vi "findRangeBearing.vi"(9 "X":dbl[](array[numeric]), 10 "ly":dbl, 11 "lx":dbl) -> (2 "tt":dbl, 3 "rr":dbl)   [LabVIEW 2009, in "LV_SLAM.lvlib"]
uses:
  LV_SLAM.lvlib
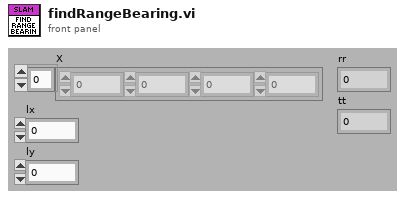
[diagram p1: front panel]
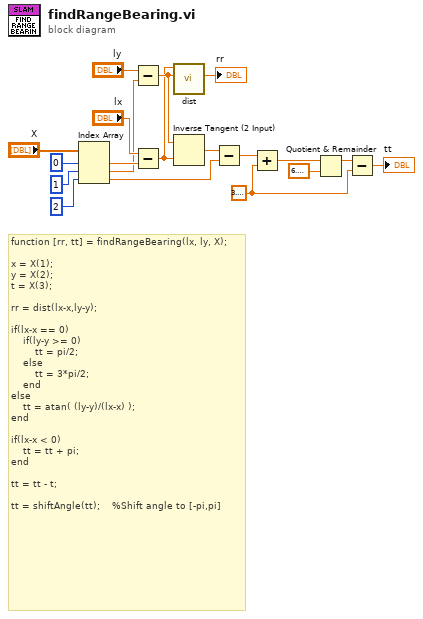
[diagram p0: block diagram]
diagram:
  w2 = 3.141592653589793
  # "function [rr, tt] = findRangeBearing(lx, ly, X);\n\nx = X(1);\ny = X(2);\nt = X(3);\n\nrr = dist(lx-x,ly-y);\n\nif(lx-x == 0)\n    if(ly-y >= 0)\n        tt = pi/2;\n    else\n        tt = 3*pi/2;\n    end\nelse\n    tt = atan( (ly-y)/(lx-x) );\nend\n\nif(lx-x < 0)\n    tt = tt + pi;\nend\n\ntt = tt - t;    \n\ntt = shiftAngle(tt);    %Shift angle to [-pi,pi]"
  n1 = Index Array(array="X", index #1=0 ("index"), index #2=1 ("index"), index #3=2 ("index")) -> (element #1=w14:dbl, element #2=w12:dbl, element #3=w7:dbl)
  n2 = Subtract(x="ly", y=w12) -> (x-y=w10:dbl)
  n3 = Subtract(x="lx", y=w14) -> (x-y=w9:dbl)
  n4 = call "dist.vi"("y"=w10, "x"=w9) -> ("d"=→"rr":dbl)  [unwired: 9 in]
  n5 = Inverse Tangent (2 Input)(1:w9, 2:w10) -> (0:w8:dbl)
  n6 = Subtract(x=w8, y=w7) -> (x-y=w6:dbl)
  n7 = Add(x=w6, y=w2) -> (x+y=w5:dbl)
  n8 = Quotient & Remainder(x=w5, y=6.283185307179586) -> (x-y*floor(x/y)=w3:dbl)  [unwired: 1 out]
  n9 = Subtract(x=w3, y=w2) -> (x-y=→"tt":dbl)
